vi "Rinocloud_csv_data_upload.vi"(3 "local storage":T2={"Store locally"=TRUE, "ancestor array"=[], "Store metadata"=TRUE}, 4 "Parent ID":string="name", 5 "Extra metadata array":T4(array[cluster])=[{"Attribute"="", "Value"="", "Data type"=enum."<null>"}], 6 "Notes":string, 7 "Tags":string, 8 "error in (no error)":errorcluster, 9 "2D numerical data":dbl[][](array[numeric]) format="%0.2f", 10 "1D numerical data":dbl[](array[numeric]) format="%0.2f", 11 "Name":string) -> (0 "error out":errorcluster, 1 "Status":T3={"headers"="", "body"="", "ID"="", "Saved"=TRUE})   [LabVIEW 2013, in "Rinocloud Library.lvlib"]
uses:
  Rinocloud Library.lvlib
  <vilib>/Utility/file.llb/Write To Spreadsheet File (DBL).vi
panel:
  in  "ancestor array":T1(array[cluster])
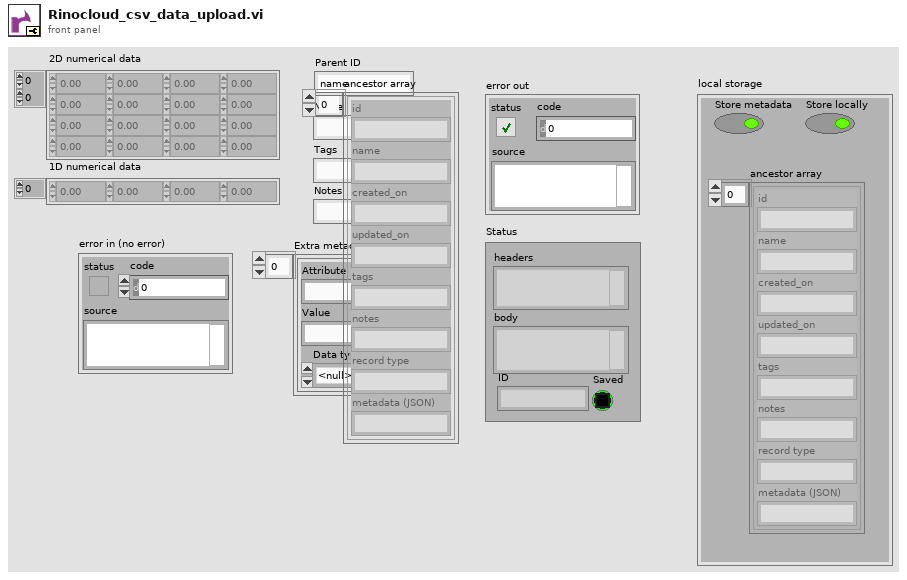
[diagram p1: front panel]
types:
  T1 = cluster{"id":string, "name":string, "created_on":string, "updated_on":string, "tags":string, "notes":string, "record type":string, "metadata (JSON)":string}[]
  T2 = cluster{"Store locally":bool, "ancestor array":cluster{"id":string, "name":string, "created_on":string, "updated_on":string, "tags":string, "notes":string, "record type":string, "metadata (JSON)":string}[], "Store metadata":bool}
  T3 = cluster{"headers":string, "body":string, "ID":string, "Saved":bool}
  T4 = cluster{"Attribute":string, "Value":string, "Data type":enum16{"Numeric", "String", "1D array of strings", "1D array of doubles", "Data JSON string", "<null>"}}[]
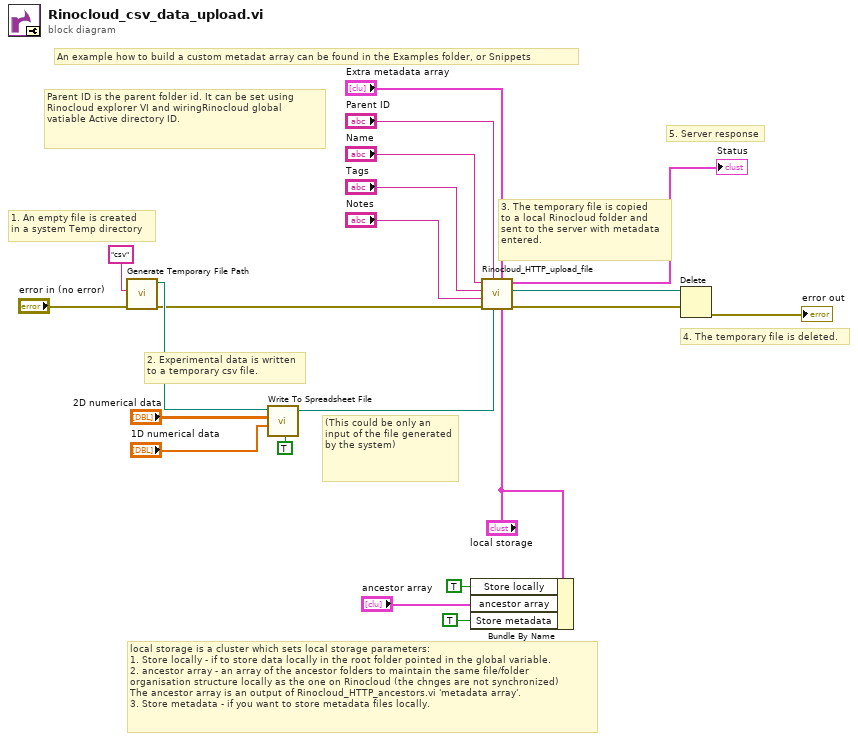
[diagram p0: block diagram]
diagram:
  # "local storage is a cluster which sets local storage parameters:\n1. Store locally - if to store data locally in the root folder pointed in the global variable.\n2. ancestor array - an array of the ancestor folders to maintain the same file/folder \norganisation structure locally as the one on Rinocloud (the chnges are not synchronized)\nThe ancestor array is an output of Rinocloud_HTTP_ancestors.vi 'metadata array'.\n3. Store metadata - if you want to store metadata files locally."
  # "(This could be only an input of the file generated by the system)"
  # "Parent ID is the parent folder id. It can be set using Rinocloud explorer VI and wiringRinocloud global vatiable Active directory ID."
  # "An example how to build a custom metadat array can be found in the Examples folder, or Snippets"
  # "5. Server response"
  # "4. The temporary file is deleted."
  # "3. The temporary file is copied\nto a local Rinocloud folder and\nsent to the server with metadata\nentered."
  # "2. Experimental data is written\nto a temporary csv file."
  # "1. An empty file is created\nin a system Temp directory"
  n1 = call <vilib>:"Generate Temporary File Path.vi"("error in (no error)"="error in (no error)", "Temporary File Extension (tmp)"="csv" ("name or relative path")) -> ("error out"=w7:errorcluster, "Unique Temporary File Path"=w19:path)  [unwired: 8 in]
  n2 = call-poly <vilib>:"Write To Spreadsheet File.vi"("transpose? (no:F)"=TRUE, "1D data"="1D numerical data", "2D data"="2D numerical data", "file path (dialog if empty)"=w19) -> ("new file path (Not A Path if cancelled)"=w14:path)  [unwired: 4 in]
  n3 = Bundle By Name(cluster="local storage", "Store locally"=TRUE, "ancestor array"="ancestor array", "Store metadata"=TRUE) -> ()  [unwired: 1 out]
  n4 = call "Rinocloud_HTTP_upload_file.vi"("local storage"="local storage", "Extra metadata array"="Extra metadata array", "Path in"=w14, "Parent ID"="Parent ID", "error in (no error)"=w7, "Notes"="Notes", "Tags"="Tags", "Name"="Name") -> ("error out"=w6:errorcluster, "Path out"=w15:path, "Status"=→"Status":T3)  [unwired: 1 in]
  n5 = Delete(path (use dialog)=w15, error in=w6) -> (error out=→"error out":errorcluster)  [unwired: 3 in, 2 out]
